vi "02 HEWH Stand Overide.vi"() -> ()   [LabVIEW 2012]
uses:
  EquipReferences.ctl
  HEWH Tank Indicator.ctl
  Intellifaucet/Intellfaucet Mode.ctl
  PowerElements.ctl
  Use Modes.ctl
  <vilib>/Platform/fileVersionInfo.llb/FileVersionInformation.ctl
  GEA2/HEWH_Mode.ctl
  ValveBankPositions.ctl
  ChannelSettings.ctl
  Global HEWH.vi
  <vilib>/Utility/file.llb/Write To Spreadsheet File (string).vi
panel:
  in  "GEA2 Max Retry":i32
  in  "Valve Set D":T1
  in  "Valve Set C":T1
  in  "Valve Set B":T1
  in  "Valve Set A":T1
  out "Source Array":string[](array[string])
  out "Pannel List":string[](array[string])
  in  "GEA2?":bool=TRUE
  out "Data Array":string[][](array[string])
  out "FileVersionInfo Out":T2
  out "Computer Name":string
  out "Label Array":string[](array[string])
  out "Chanel List":string
  in  "Serial Data In":string
  out "RLT":bool
  in  "Out VLV D":enum8{"CLOSE", "OPEN"}(ring)=enum."OPEN"
  in  "Drain VLV D":enum8{"OPEN", "CLOSE"}(ring)=enum."CLOSE"
  in  "In VLV D":enum8{"OPEN", "CLOSE"}(ring)=enum."CLOSE"
  in  "Out VLV C":enum8{"CLOSE", "OPEN"}(ring)=enum."OPEN"
  in  "Drain VLV C":enum8{"OPEN", "CLOSE"}(ring)=enum."CLOSE"
  in  "In VLV C":enum8{"OPEN", "CLOSE"}(ring)=enum."CLOSE"
  in  "Out VLV B":enum8{"CLOSE", "OPEN"}(ring)=enum."OPEN"
  in  "Drain VLV B":enum8{"OPEN", "CLOSE"}(ring)=enum."CLOSE"
  in  "In VLV B":enum8{"OPEN", "CLOSE"}(ring)=enum."CLOSE"
  out "IP Add":string
  out "BUG array":string[](array[string])
  in  "Data File Directory":path=path "c:/data"
  out "Ver.":string="Development"
  in  "COM Port":refnum<visa-resource-name>="COM3"
  in  "DRM Mode Setting":T3=3 items=["CRITICAL", "HIGH", "MEDIUM", "Normal"]
  in  "Equipment":T4={"COM Port"="COM3", "MW100"="MW100", "AG34970"="A-34972A", "Chamber"="WT500"}
  out "MW100":refnum<visa-resource-name>
  out "Local?":bool=TRUE
  in  "Help":bool
  in  "Out VLV":enum8{"CLOSE", "OPEN"}(ring)=enum."OPEN"
  in  "Drain VLV":enum8{"OPEN", "CLOSE"}(ring)=enum."CLOSE"
  in  "In VLV":enum8{"OPEN", "CLOSE"}(ring)=enum."CLOSE"
  out "Error Out":errorcluster
  out "Ready":bool
  in  "Stop Test":bool
  in  "HEWH Power":bool
  in  "Semiphore":T5=refnum
  in  "Safe Mode":bool=TRUE
  in  "Expansion Tank?":bool=TRUE
  in  "IF Stop":bool
  in  "IF Start":bool
  in  "IFaucet Driver":bool
  in  "Percent Flow":dbl(slide)=100.0 scale=0.0..100.0
  in  "Temperature(F)":dbl(slide)=58.0 scale=40.0..120.0
  in  "Mode":T6
  in  "Error In":errorcluster
  out "Update Mode":bool=TRUE
  in  "SetPoint":u8=130
  out "Stop Err":errorcluster
  out "IF Error":errorcluster
  out "kW":dbl
  in  "GEA2 Mode Read":T7=enum."Vacation"
  out "Serial Port Error":errorcluster
  in  "Reset Count":bool
  in  "P-H":bool
  out "Use Agilent?":bool
  out "Gather Data Error":errorcluster
  out "Header?":bool=TRUE
  out "Voltage Reading":dbl=240.0
  in  "Sample Period (S)":dbl=10.0
  out "POWER":T8
  out "Serial Port Available?":bool=TRUE
  in  "Write To File":bool
  out "file path (dialog if empty)":path=path "c:/data/20110112-2122_HEWH-MAN_OV.csv"
  out "WriteDataCount":i32
  out "DATA - Label, Value, Source":string[][](array[string])
  out "Tank Display":T9 {"TC6" format="%.2g"; "TIN" format="%.2g"; "TOUT" format="%.2g"; "Mean" format="%.2f"; "Std Dev" format="%.2f"; "TC5" format="%.2g"; "TC4" format="%.2g"; "TC3" format="%.2g"; "TC2" format="%.2g"; "TC1" format="%.2g"}
  in  "Termperature":dbl=58.0 format="%_6g"
  in  "Read Flow":bool=TRUE
  out "Pulse":i32
  in  "Flow Totalizer Control":bool=TRUE
  out "Dispensed":dbl
  out "ToutMin":dbl
  out "ToutMax":dbl
  in  "Gallon Target":dbl=10.72
  in  "GPM Target":dbl=3.0
  in  "Dispense":bool
  out "LBS":dbl
  in  "Reset Totalizer":bool
  out "Gallons":dbl
  out "Flow Meter":dbl(graph)
  # "HEWH Test Stand Overide"
  # "Intellifaucet Control"
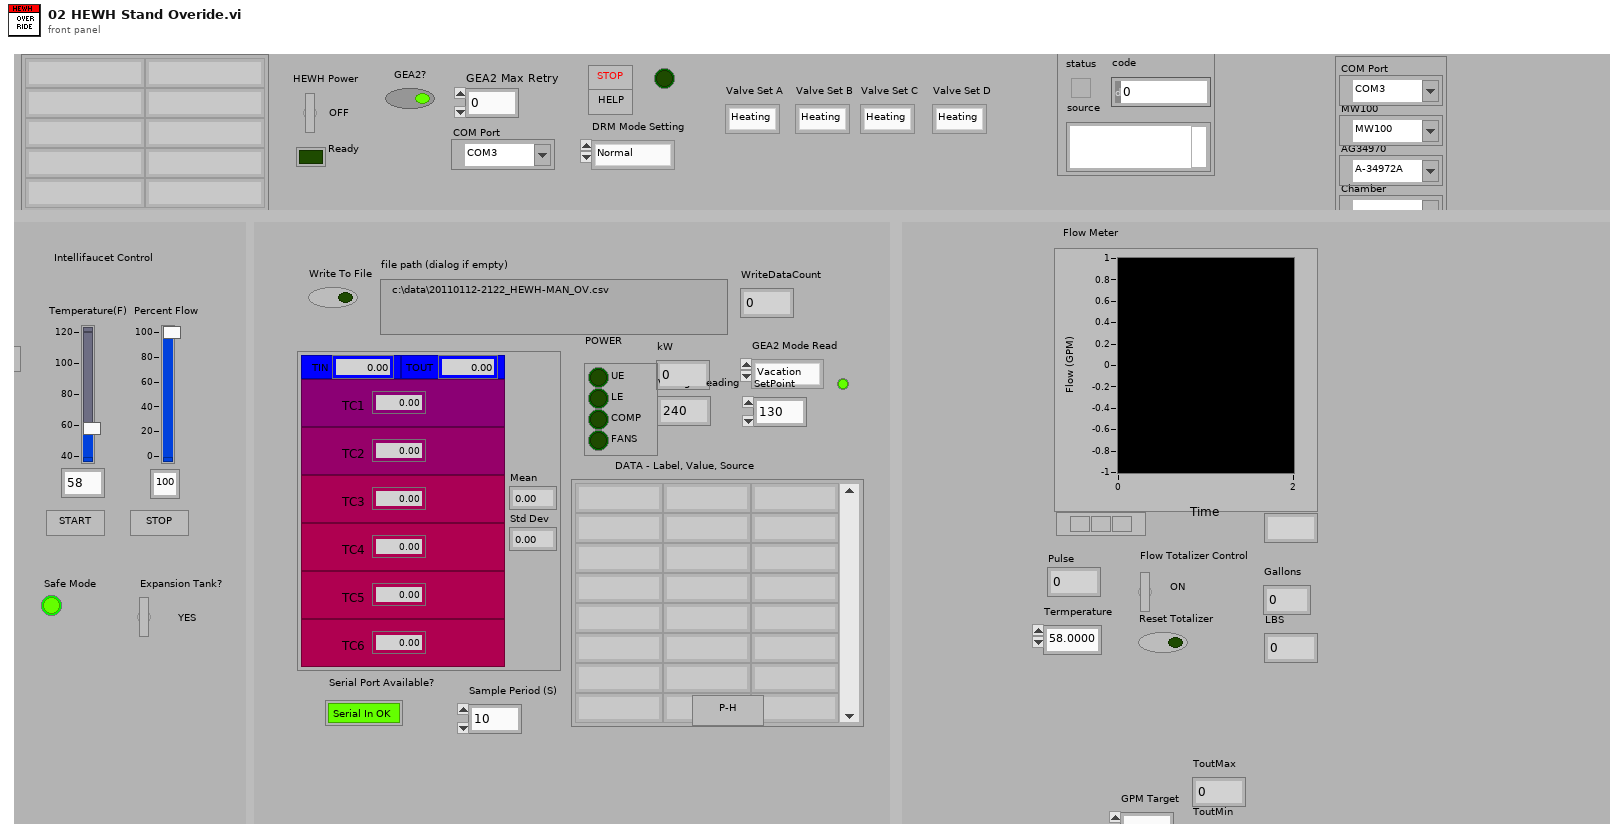
[diagram p1: front panel]
types:
  T1 = typedef "ValveBankPositions.ctl" = enum16{"Heating", "Purge", "Resting", "Draw"}
  T2 = typedef "FileVersionInformation.ctl" = cluster{"FileVersion":string, "ProductName":string, "InternalName":string, "CompanyName":string, "LegalCopyright":string, "FileDescription":string}
  T3 = typedef "Use Modes.ctl" = u16
  T4 = typedef "EquipReferences.ctl" = cluster{"COM Port":refnum<visa-resource-name>, "MW100":refnum<visa-resource-name>, "AG34970":refnum<visa-resource-name>, "Chamber":refnum<visa-resource-name>}
  T5 = typedef "Semaphore RefNum" = refnum<k1>
  T6 = typedef "Intellfaucet Mode.ctl" = enum16{"Adjust Temp", "Adjust Flow", "Start Flow", "Stop Flow"}
  T7 = typedef "HEWH_Mode.ctl" = enum16{"Hybrid", "StdElectric", "eHeat", "HighDemand", "Vacation"}
  T8 = typedef "PowerElements.ctl" = cluster{"UE":bool, "LE":bool, "COMP":bool, "FANS":bool}
  T9 = typedef "HEWH Tank Indicator.ctl" = cluster{"TC1-D":bool, "TC2-D":bool, "TC3-D":bool, "TC4-D":bool, "TC5-D":bool, "RTD_IN":bool, "RTDOUT":bool, "TC1":dbl, "TC2":dbl, "TC3":dbl, "TC4":dbl, "TC5":dbl, "TIN":dbl, "TOUT":dbl, "Std Dev":dbl, "Mean":dbl, "TC6-D":bool, "TC6":dbl}
  T10 = typedef "ChannelSettings.ctl" = u32
  T11 = enum16{"Computation Start", "Computation stop", "Reset Computation", "Clear Computation"}
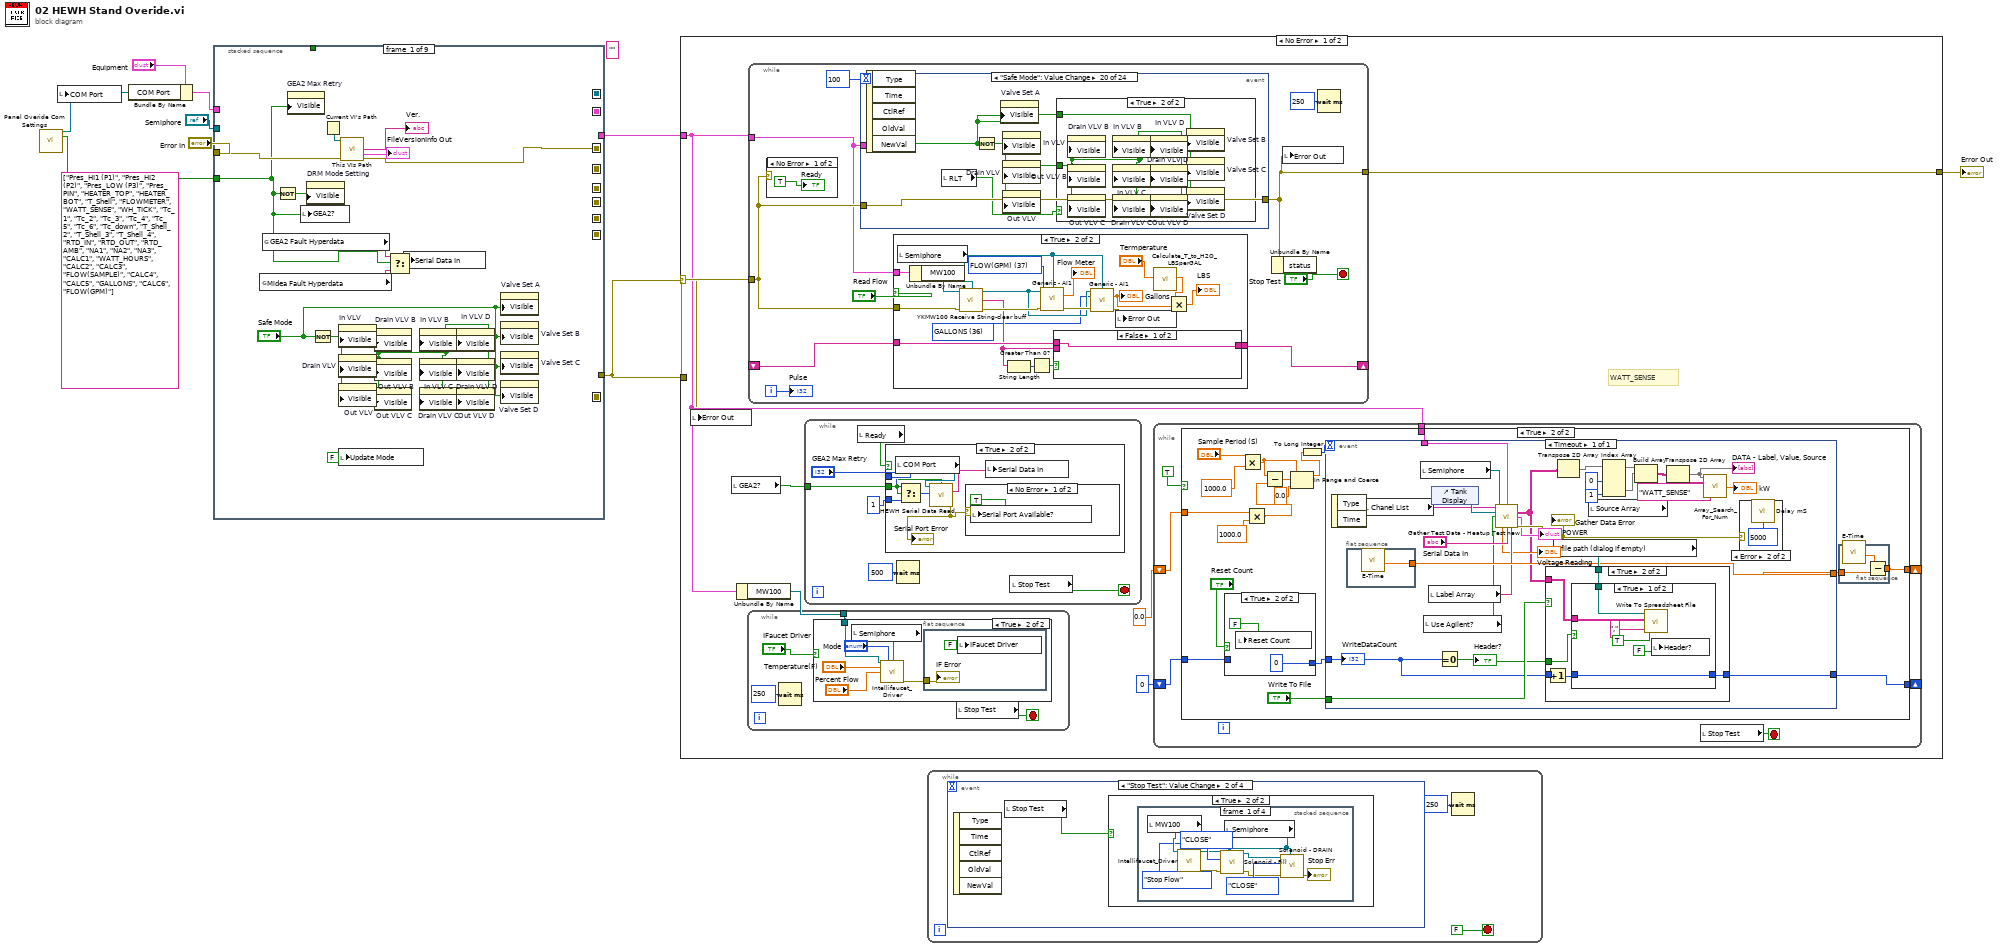
[diagram p0: block diagram]
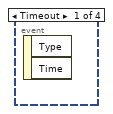
[diagram p2: hidden frame]
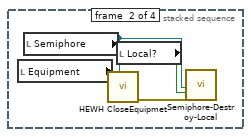
[diagram p4: hidden frame]
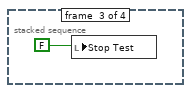
[diagram p5: hidden frame]
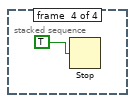
[diagram p6: hidden frame]
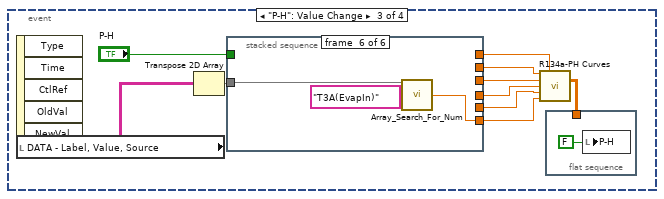
[diagram p7: hidden frame]
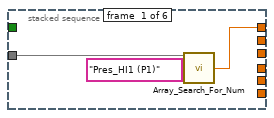
[diagram p8: hidden frame]
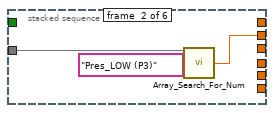
[diagram p9: hidden frame]
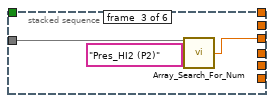
[diagram p10: hidden frame]
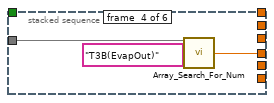
[diagram p11: hidden frame]
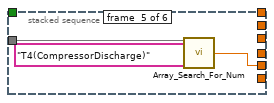
[diagram p12: hidden frame]
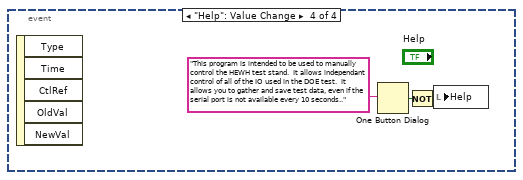
[diagram p13: hidden frame]
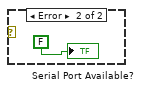
[diagram p15: hidden frame]
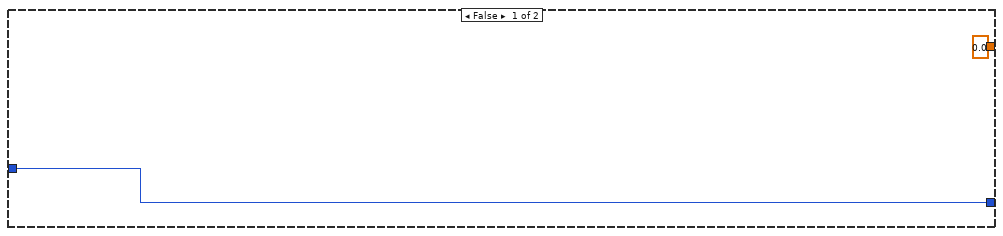
[diagram p17: hidden frame]
diagram:
  (unwired) "" ("Label.Text")
  (unwired) string[] ["Pres_HI1 (P1)", "Pres_HI2 (P2)", "Pres_LOW (P3)", "Pres_PIN", "HEATER_TOP", "HEATER_BOT", "T_Shell", "FLOWMETER", "WATT_SENSE", "WH_TICK", "Tc_1", "Tc_2", "Tc_3", "Tc_4", "Tc_5", "Tc_6", "Tc_down", "T_Shell_2", "T_Shell_3", "T_Shell_4", "RTD_IN", "RTD_OUT", "RTD_AMB", "NA1", "NA2", "NA3", "CALC1", "WATT_HOURS", "CALC2", "CALC3", "FLOW(SAMPLE)", "CALC4", "CALC5", "GALLONS", "CALC6", "FLOW(GPM)"] ("output array")
  n1 = call "Panel Overide Com Settings.vi"() -> ("COM Port Out"=w1:refnum<visa-resource-name>, "GEA2 HyperData Out"=w2:bool)  [unwired: 14 in]
  n2 = local write "COM Port"(w1) -> ()
  n3 = Bundle By Name(cluster="Equipment", "COM Port"=w1) -> (w4:T4)
  n4 = stacked-sequence {
    seq-local: [_ _ w45 _ _ _ _ _ _] -> [_ _ _ w77 _ _ _ _ _]
    seq-local: [_ _ w41 _ _ _ _ _ _] -> [_ _ _ w64 w93 w115 w129 _ _]
    seq-local: [w19 _ _ _ _ _ _ _ _] -> [_ w27 _ _ _ _ _ _ _]
    seq-local: [_ w34 _ _ _ _ _ _ _] -> [_ _ w38 _ _ _ _ _ _]
    seq-local: [_ _ _ w61 _ _ _ _ _] -> [_ _ _ _ w88 _ _ _ _]
    seq-local: [_ _ _ _ w89 _ _ _ _] -> [_ _ _ _ _ w107 _ _ _]
    seq-local: [_ _ _ _ _ w108 _ _ _] -> [_ _ _ _ _ _ w130 _ _]
    seq-local: [_ _ _ _ _ _ w132 _ _] -> [_ _ _ _ _ _ _ w158 _]
    seq-local: [_ _ w37 _ _ _ _ _ _] -> [_ _ _ w60 w87 w106 w128 w157 w175]
    tunnel: "Error In" -> [w20 _ _ _ _ _ _ _ _]
    tunnel: w4 -> [_ _ w46 _ _ _ _ _ _]
    tunnel: [_ _ w37 _ _ _ _ _ _] -> w8
    tunnel: [_ _ _ _ _ _ _ w155 _] -> w7
    tunnel: [_ _ w40 _ _ _ _ _ _] -> _
    tunnel: "Semiphore" -> [_ _ w43 _ _ _ _ _ _]
    tunnel: w2 -> [w10 _ _ _ _ _ _ _ _]
    frame #0 {
      n5 = global read "Global HEWH.vi" "Midea Fault Hyperdata"() -> (w15:string)
      n6 = global read "Global HEWH.vi" "GEA2 Fault Hyperdata"() -> (w16:string)
      n7 = Not(x=w10) -> (.not. x?=w11:bool)
      n8 = property on="GEA2 Max Retry" class="DigNum (strict)"("Visible"=w10) -> ()  [unwired: 2 in, 2 out]
      n9 = local write "GEA2?"(w10) -> ()
      n10 = property on="DRM Mode Setting" class="Ring (strict)"("Visible"=w11) -> ()  [unwired: 2 in, 2 out]
      n11 = Not(x="Safe Mode") -> (.not. x?=w14:bool)
      n12 = Current VI's Path() -> (path=w22:path)
      n13 = local write "Update Mode"(FALSE ("Update Mode")) -> ()
      n14 = property on="In VLV" class="Enum (strict)"("Visible"=w14) -> ()  [unwired: 2 in, 2 out]
      n15 = property on="Drain VLV" class="Enum (strict)"("Visible"=w14) -> ()  [unwired: 2 in, 2 out]
      n16 = property on="Out VLV" class="Enum (strict)"("Visible"=w14) -> ()  [unwired: 2 in, 2 out]
      n17 = call "This VIs Path.vi"("path"=w22, "error in (no error)"=w20) -> ("File Version Info"=→"Ver.":string, "FileVersionInfo Out"=→"FileVersionInfo Out":T2, "error out"=w19:errorcluster)  [unwired: 9 in, 2 out]
      n18 = property on="Drain VLV B" class="Enum (strict)"("Visible"=w14) -> ()  [unwired: 2 in, 2 out]
      n19 = property on="Out VLV B" class="Enum (strict)"("Visible"=w14) -> ()  [unwired: 2 in, 2 out]
      n20 = property on="Out VLV C" class="Enum (strict)"("Visible"=w14) -> ()  [unwired: 2 in, 2 out]
      n21 = Select(t=w16, s=w10, f=w15) -> (s? t:f=w17:string)
      n22 = local write "Serial Data In"(w17) -> ()
      n23 = property on="In VLV B" class="Enum (strict)"("Visible"=w14) -> ()  [unwired: 2 in, 2 out]
      n24 = property on="In VLV C" class="Enum (strict)"("Visible"=w14) -> ()  [unwired: 2 in, 2 out]
      n25 = property on="Drain VLV C" class="Enum (strict)"("Visible"=w14) -> ()  [unwired: 2 in, 2 out]
      n26 = property on="In VLV D" class="Enum (strict)"("Visible"=w14) -> ()  [unwired: 2 in, 2 out]
      n27 = property on="Drain VLV D" class="Enum (strict)"("Visible"=w14) -> ()  [unwired: 2 in, 2 out]
      n28 = property on="Out VLV D" class="Enum (strict)"("Visible"=w14) -> ()  [unwired: 2 in, 2 out]
      n29 = property on="Valve Set A" class="Enum (strict)"("Visible"="Safe Mode") -> ()  [unwired: 2 in, 2 out]
      n30 = property on="Valve Set B" class="Enum (strict)"("Visible"="Safe Mode") -> ()  [unwired: 2 in, 2 out]
      n31 = property on="Valve Set C" class="Enum (strict)"("Visible"="Safe Mode") -> ()  [unwired: 2 in, 2 out]
      n32 = property on="Valve Set D" class="Enum (strict)"("Visible"="Safe Mode") -> ()  [unwired: 2 in, 2 out]
    }
    frame #1 {
      w33 = TRUE ("Reset")
      n33 = local read "FileVersionInfo Out"() -> (w31:T2)
      n34 = call "IP and Computer Name.vi"() -> ("Computer Name"=w32:string)  [unwired: 10 in, 1 out]
      "Computer Name" <- w32
      n35 = Unbundle By Name(w31) -> ("FileVersion"=w30:string)  [unwired: 1 out]
      n36 = call "Data_File_Init.vi"("Data File Directory"="Data File Directory", "Test_Name In:"="MANOV", "Version In:"=w30, "Computer Name In:"=w32, "error in (no error)"=w27, "File Extension:"="csv") -> ("FileName"=→"file path (dialog if empty)":path, "Data Array"=→"Data Array":string[][], "error out"=w28:errorcluster)  [unwired: 7 in]
      n37 = local write "Header?"(w33) -> ()
      n38 = call "E-Time.vi"("error in (no error)"=w28, "Reset"=w33) -> ("error out"=w34:errorcluster)  [unwired: 7 in, 2 out]
    }
    frame #2 {
      w36 = FALSE ("Visible")
      n39 = call "Semiphore-Create-Local.vi"("Semiphore"=w43, "error in (no error)"=w38, "name (unnamed)"="MW100") -> ("semaphore"=w41:T5, "Local?"=w40:bool, "error out"=w44:errorcluster)  [unwired: 14 in]
      "Local?" <- w40
      n40 = local write "Dispense"(w36) -> ()
      n41 = property on="BUG array" class="Arr (strict)"("Visible"=w36) -> ()  [unwired: 2 in, 2 out]
      n42 = local write "P-H"(w36) -> ()
      n43 = local write "Semiphore"(w41) -> ()
      n44 = case shown="True" TRUE {
        tunnel: w44 -> [w48 w56]
        tunnel: [w48 w55] -> w45
        tunnel: w46 -> [w47 w54]
        tunnel: [w47 w49] -> w37
        tunnel: w41 -> [_ w52]
        frame False {
        }
        frame True {
          n45 = call "HEWH InitializeEquipmet.vi"("Semiphore"=w52, "Error In"=w56, "Equipment"=w54) -> ("Error Out"=w55:errorcluster, "LAN IP Address"=→"IP Add":string, "Equipment Out"=w49:T4)  [unwired: 5 in, 1 out]
          n46 = local write "Ready"(FALSE ("Ready")) -> ()
          n47 = Unbundle(w49) -> ("MW100"=→"MW100":refnum<visa-resource-name>)  [unwired: 3 out]
          n48 = local write "Equipment"(w49) -> ()
        }
      }
      n49 = local write "Reset Totalizer"(w36) -> ()
      "Tank Display" <- T9 {"TC1-D"=FALSE, "TC2-D"=FALSE, "TC3-D"=FALSE, "TC4-D"=FALSE, "TC5-D"=FALSE, "RTD_IN"=FALSE, "RTDOUT"=FALSE, "TC1"=0.0, "TC2"=0.0, "TC3"=0.0, "TC4"=0.0, "TC5"=0.0, "TIN"=0.0, "TOUT"=0.0, "Std Dev"=0.0, "Mean"=0.0, "TC6-D"=FALSE, "TC6"=0.0} ("Tank Display")
    }
    frame #3 {
      w65 = FALSE ("Stop Test")
      w69 = T10 30 items=["4-20_OUT", "Pres_HI1", "Pres_HI2", "Pres_LOW", "Pres_PIN", "HEATER_TOP", "HEATER_BOT", "T_Shell", "FLOWMETER", "WATT_SENSE", "WH_TICK", "Tc_1", "Tc_2", "Tc_3", "Tc_4", "Tc_5", "Tc_6", "Tc_down", "T_Shell_2", "T_Shell_3", "T_Shell_4", "RTD_IN", "RTD_OUT", "RTD_AMB", "INTF_TEMPFLO", "INTF_READY", "INTF_START", "INTF_STOP", "DRM_LOW", "DRM_HIGH", "PWR_MAIN", "VLV_DUMP", "VLV_OUT", "VLV_IN", "WATT_HOURS", "FLOW(SAMPLE)", "GALLONS", "FLOW(GPM)"] ("Channel_Enum")
      w70 = T10 33 items=["4-20_OUT", "Pres_HI1", "Pres_HI2", "Pres_LOW", "Pres_PIN", "HEATER_TOP", "HEATER_BOT", "T_Shell", "FLOWMETER", "WATT_SENSE", "WH_TICK", "Tc_1", "Tc_2", "Tc_3", "Tc_4", "Tc_5", "Tc_6", "Tc_down", "T_Shell_2", "T_Shell_3", "T_Shell_4", "RTD_IN", "RTD_OUT", "RTD_AMB", "INTF_TEMPFLO", "INTF_READY", "INTF_START", "INTF_STOP", "DRM_LOW", "DRM_HIGH", "PWR_MAIN", "VLV_DUMP", "VLV_OUT", "VLV_IN", "WATT_HOURS", "FLOW(SAMPLE)", "GALLONS", "FLOW(GPM)"] ("Channel_Enum")
      w71 = T10 32 items=["4-20_OUT", "Pres_HI1", "Pres_HI2", "Pres_LOW", "Pres_PIN", "HEATER_TOP", "HEATER_BOT", "T_Shell", "FLOWMETER", "WATT_SENSE", "WH_TICK", "Tc_1", "Tc_2", "Tc_3", "Tc_4", "Tc_5", "Tc_6", "Tc_down", "T_Shell_2", "T_Shell_3", "T_Shell_4", "RTD_IN", "RTD_OUT", "RTD_AMB", "INTF_TEMPFLO", "INTF_READY", "INTF_START", "INTF_STOP", "DRM_LOW", "DRM_HIGH", "PWR_MAIN", "VLV_DUMP", "VLV_OUT", "VLV_IN", "WATT_HOURS", "FLOW(SAMPLE)", "GALLONS", "FLOW(GPM)"] ("Channel_Enum")
      w73 = T10 31 items=["4-20_OUT", "Pres_HI1", "Pres_HI2", "Pres_LOW", "Pres_PIN", "HEATER_TOP", "HEATER_BOT", "T_Shell", "FLOWMETER", "WATT_SENSE", "WH_TICK", "Tc_1", "Tc_2", "Tc_3", "Tc_4", "Tc_5", "Tc_6", "Tc_down", "T_Shell_2", "T_Shell_3", "T_Shell_4", "RTD_IN", "RTD_OUT", "RTD_AMB", "INTF_TEMPFLO", "INTF_READY", "INTF_START", "INTF_STOP", "DRM_LOW", "DRM_HIGH", "PWR_MAIN", "VLV_DUMP", "VLV_OUT", "VLV_IN", "WATT_HOURS", "FLOW(SAMPLE)", "GALLONS", "FLOW(GPM)"] ("Channel_Enum")
      n50 = local read "Safe Mode"() -> (w58:bool)
      n51 = Unbundle By Name(w60) -> ("MW100"=w72:refnum<visa-resource-name>)
      n52 = local write "IFaucet Driver"(w65) -> ()
      n53 = local write "Stop Test"(w65) -> ()
      n54 = local write "Ready"(w65) -> ()
      n55 = call "YKMW100 VF0 Relay Status.vi"("VISA session"=w72, "Semiphore"=w64, "Channel_Enum"=w69, "error in (no error)"=w77) -> ("Output On"=w62:bool, "DO Card in Slot 5"=w59:bool, "error out"=w76:errorcluster)  [unwired: 8 in, 1 out]
      "RLT" <- w59
      n56 = call "YKMW100 VF0 Relay Status.vi"("VISA session"=w72, "Semiphore"=w64, "Channel_Enum"=w70, "error in (no error)"=w76) -> ("Output On"=w68:bool, "error out"=w75:errorcluster)  [unwired: 8 in, 2 out]
      n57 = call "YKMW100 VF0 Relay Status.vi"("VISA session"=w72, "Semiphore"=w64, "Channel_Enum"=w71, "error in (no error)"=w75) -> ("Output On"=w67:bool, "error out"=w74:errorcluster)  [unwired: 8 in, 2 out]
      n58 = call "YKMW100 VF0 Relay Status.vi"("VISA session"=w72, "Semiphore"=w64, "Channel_Enum"=w73, "error in (no error)"=w74) -> ("Output On"=w66:bool, "error out"=w61:errorcluster)  [unwired: 8 in, 2 out]
      n59 = Not(x=w58) -> (.not. x?=w57:bool)
      n60 = case shown="False" w59 {
        tunnel: w57 -> [w79 _]
        tunnel: w58 -> [w78 _]
        frame True {
          n61 = property on="Drain VLV B" class="Enum (strict)"("Visible"=w79) -> ()  [unwired: 2 in, 2 out]
          n62 = property on="Out VLV B" class="Enum (strict)"("Visible"=w79) -> ()  [unwired: 2 in, 2 out]
          n63 = property on="Out VLV C" class="Enum (strict)"("Visible"=w79) -> ()  [unwired: 2 in, 2 out]
          n64 = property on="In VLV B" class="Enum (strict)"("Visible"=w79) -> ()  [unwired: 2 in, 2 out]
          n65 = property on="In VLV C" class="Enum (strict)"("Visible"=w79) -> ()  [unwired: 2 in, 2 out]
          n66 = property on="Drain VLV C" class="Enum (strict)"("Visible"=w79) -> ()  [unwired: 2 in, 2 out]
          n67 = property on="In VLV D" class="Enum (strict)"("Visible"=w79) -> ()  [unwired: 2 in, 2 out]
          n68 = property on="Drain VLV D" class="Enum (strict)"("Visible"=w79) -> ()  [unwired: 2 in, 2 out]
          n69 = property on="Out VLV D" class="Enum (strict)"("Visible"=w79) -> ()  [unwired: 2 in, 2 out]
          n70 = property on="Valve Set B" class="Enum (strict)"("Visible"=w78) -> ()  [unwired: 2 in, 2 out]
          n71 = property on="Valve Set C" class="Enum (strict)"("Visible"=w78) -> ()  [unwired: 2 in, 2 out]
          n72 = property on="Valve Set D" class="Enum (strict)"("Visible"=w78) -> ()  [unwired: 2 in, 2 out]
        }
        frame False {
          w80 = FALSE ("Visible")
          n73 = property on="Drain VLV B" class="Enum (strict)"("Visible"=w80) -> ()  [unwired: 2 in, 2 out]
          n74 = property on="Out VLV B" class="Enum (strict)"("Visible"=w80) -> ()  [unwired: 2 in, 2 out]
          n75 = property on="Out VLV C" class="Enum (strict)"("Visible"=w80) -> ()  [unwired: 2 in, 2 out]
          n76 = property on="In VLV B" class="Enum (strict)"("Visible"=w80) -> ()  [unwired: 2 in, 2 out]
          n77 = property on="In VLV C" class="Enum (strict)"("Visible"=w80) -> ()  [unwired: 2 in, 2 out]
          n78 = property on="Drain VLV C" class="Enum (strict)"("Visible"=w80) -> ()  [unwired: 2 in, 2 out]
          n79 = property on="In VLV D" class="Enum (strict)"("Visible"=w80) -> ()  [unwired: 2 in, 2 out]
          n80 = property on="Drain VLV D" class="Enum (strict)"("Visible"=w80) -> ()  [unwired: 2 in, 2 out]
          n81 = property on="Out VLV D" class="Enum (strict)"("Visible"=w80) -> ()  [unwired: 2 in, 2 out]
          n82 = property on="Valve Set B" class="Enum (strict)"("Visible"=w80) -> ()  [unwired: 2 in, 2 out]
          n83 = property on="Valve Set C" class="Enum (strict)"("Visible"=w80) -> ()  [unwired: 2 in, 2 out]
          n84 = property on="Valve Set D" class="Enum (strict)"("Visible"=w80) -> ()  [unwired: 2 in, 2 out]
        }
      }
      n85 = Not(x=w62) -> (.not. x?=w63:bool)
      n86 = case shown="False" w68 {
        frame True {
          n87 = local write "In VLV"(enum8{"OPEN", "CLOSE"}."CLOSE" ("INPUT VALVE")) -> ()
        }
        frame False {
          n88 = local write "In VLV"(enum8{"OPEN", "CLOSE"}."OPEN" ("INPUT VALVE")) -> ()
        }
      }
      n89 = case shown="False" w66 {
        frame True {
          n90 = local write "Drain VLV"(enum8{"OPEN", "CLOSE"}."OPEN" ("DRAIN VALVE")) -> ()
        }
        frame False {
          n91 = local write "Drain VLV"(enum8{"OPEN", "CLOSE"}."CLOSE" ("DRAIN VALVE")) -> ()
        }
      }
      n92 = case shown="False" w67 {
        frame True {
          n93 = local write "Out VLV"(enum8{"CLOSE", "OPEN"}."CLOSE" ("VALVE OUT")) -> ()
        }
        frame False {
          n94 = local write "Out VLV"(enum8{"CLOSE", "OPEN"}."OPEN" ("VALVE OUT")) -> ()
        }
      }
      n95 = local write "HEWH Power"(w63) -> ()
      n96 = property on="RLT" class="Bool (strict)"("Val(Sgnl)"=w59) -> ()  [unwired: 2 in, 2 out]
    }
    frame #4 {
      w92 = T10 41 items=["4-20_OUT", "Pres_HI1", "Pres_HI2", "Pres_LOW", "Pres_PIN", "HEATER_TOP", "HEATER_BOT", "T_Shell", "FLOWMETER", "WATT_SENSE", "WH_TICK", "Tc_1", "Tc_2", "Tc_3", "Tc_4", "Tc_5", "Tc_6", "Tc_down", "T_Shell_2", "T_Shell_3", "T_Shell_4", "RTD_IN", "RTD_OUT", "RTD_AMB", "INTF_TEMPFLO", "INTF_READY", "INTF_START", "INTF_STOP", "DRM_LOW", "DRM_HIGH", "PWR_MAIN", "VLV_DUMP", "VLV_OUT", "VLV_IN", "WATT_HOURS", "FLOW(SAMPLE)", "GALLONS", "FLOW(GPM)", "FLOW_CALC_GAIN", "FLOW_CALC_OFFSET", "FLOW_CALC_THRESHOLD", "VLV_DUMP_2", "VLV_OUT_2", "VLV_IN_2", "VLV_DUMP_3", "VLV_OUT_3", "VLV_IN_3", "VLV_DUMP_4", "VLV_OUT_4", "VLV_IN_4"] ("Channel_Enum")
      w91 = T10 42 items=["4-20_OUT", "Pres_HI1", "Pres_HI2", "Pres_LOW", "Pres_PIN", "HEATER_TOP", "HEATER_BOT", "T_Shell", "FLOWMETER", "WATT_SENSE", "WH_TICK", "Tc_1", "Tc_2", "Tc_3", "Tc_4", "Tc_5", "Tc_6", "Tc_down", "T_Shell_2", "T_Shell_3", "T_Shell_4", "RTD_IN", "RTD_OUT", "RTD_AMB", "INTF_TEMPFLO", "INTF_READY", "INTF_START", "INTF_STOP", "DRM_LOW", "DRM_HIGH", "PWR_MAIN", "VLV_DUMP", "VLV_OUT", "VLV_IN", "WATT_HOURS", "FLOW(SAMPLE)", "GALLONS", "FLOW(GPM)", "FLOW_CALC_GAIN", "FLOW_CALC_OFFSET", "FLOW_CALC_THRESHOLD", "VLV_DUMP_2", "VLV_OUT_2", "VLV_IN_2", "VLV_DUMP_3", "VLV_OUT_3", "VLV_IN_3", "VLV_DUMP_4", "VLV_OUT_4", "VLV_IN_4"] ("Channel_Enum")
      w90 = T10 43 items=["4-20_OUT", "Pres_HI1", "Pres_HI2", "Pres_LOW", "Pres_PIN", "HEATER_TOP", "HEATER_BOT", "T_Shell", "FLOWMETER", "WATT_SENSE", "WH_TICK", "Tc_1", "Tc_2", "Tc_3", "Tc_4", "Tc_5", "Tc_6", "Tc_down", "T_Shell_2", "T_Shell_3", "T_Shell_4", "RTD_IN", "RTD_OUT", "RTD_AMB", "INTF_TEMPFLO", "INTF_READY", "INTF_START", "INTF_STOP", "DRM_LOW", "DRM_HIGH", "PWR_MAIN", "VLV_DUMP", "VLV_OUT", "VLV_IN", "WATT_HOURS", "FLOW(SAMPLE)", "GALLONS", "FLOW(GPM)", "FLOW_CALC_GAIN", "FLOW_CALC_OFFSET", "FLOW_CALC_THRESHOLD", "VLV_DUMP_2", "VLV_OUT_2", "VLV_IN_2", "VLV_DUMP_3", "VLV_OUT_3", "VLV_IN_3", "VLV_DUMP_4", "VLV_OUT_4", "VLV_IN_4"] ("Channel_Enum")
      n97 = Unbundle By Name(w87) -> ("MW100"=w97:refnum<visa-resource-name>)
      n98 = call "YKMW100 VF0 Relay Status.vi"("VISA session"=w97, "Semiphore"=w93, "Channel_Enum"=w90, "error in (no error)"=w88) -> ("Output On"=w96:bool, "error out"=w99:errorcluster)  [unwired: 8 in, 2 out]
      n99 = call "YKMW100 VF0 Relay Status.vi"("VISA session"=w97, "Semiphore"=w93, "Channel_Enum"=w91, "error in (no error)"=w99) -> ("Output On"=w95:bool, "error out"=w98:errorcluster)  [unwired: 8 in, 2 out]
      n100 = call "YKMW100 VF0 Relay Status.vi"("VISA session"=w97, "Semiphore"=w93, "Channel_Enum"=w92, "error in (no error)"=w98) -> ("Output On"=w94:bool, "error out"=w89:errorcluster)  [unwired: 8 in, 2 out]
      n101 = case shown="True" w94 {
        frame True {
          n102 = local write "Drain VLV B"(enum8{"OPEN", "CLOSE"}."OPEN" ("DRAIN VALVE")) -> ()
        }
        frame False {
          n103 = local write "Drain VLV B"(enum8{"OPEN", "CLOSE"}."CLOSE" ("DRAIN VALVE")) -> ()
        }
      }
      n104 = case shown="False" w96 {
        frame True {
          n105 = local write "In VLV B"(enum8{"OPEN", "CLOSE"}."CLOSE" ("INPUT VALVE")) -> ()
        }
        frame False {
          n106 = local write "In VLV B"(enum8{"OPEN", "CLOSE"}."OPEN" ("INPUT VALVE")) -> ()
        }
      }
      n107 = case shown="True" w95 {
        frame True {
          n108 = local write "Out VLV B"(enum8{"CLOSE", "OPEN"}."CLOSE" ("VALVE OUT")) -> ()
        }
        frame False {
          n109 = local write "Out VLV B"(enum8{"CLOSE", "OPEN"}."OPEN" ("VALVE OUT")) -> ()
        }
      }
    }
    frame #5 {
      w114 = T10 44 items=["4-20_OUT", "Pres_HI1", "Pres_HI2", "Pres_LOW", "Pres_PIN", "HEATER_TOP", "HEATER_BOT", "T_Shell", "FLOWMETER", "WATT_SENSE", "WH_TICK", "Tc_1", "Tc_2", "Tc_3", "Tc_4", "Tc_5", "Tc_6", "Tc_down", "T_Shell_2", "T_Shell_3", "T_Shell_4", "RTD_IN", "RTD_OUT", "RTD_AMB", "INTF_TEMPFLO", "INTF_READY", "INTF_START", "INTF_STOP", "DRM_LOW", "DRM_HIGH", "PWR_MAIN", "VLV_DUMP", "VLV_OUT", "VLV_IN", "WATT_HOURS", "FLOW(SAMPLE)", "GALLONS", "FLOW(GPM)", "FLOW_CALC_GAIN", "FLOW_CALC_OFFSET", "FLOW_CALC_THRESHOLD", "VLV_DUMP_2", "VLV_OUT_2", "VLV_IN_2", "VLV_DUMP_3", "VLV_OUT_3", "VLV_IN_3", "VLV_DUMP_4", "VLV_OUT_4", "VLV_IN_4"] ("Channel_Enum")
      w113 = T10 45 items=["4-20_OUT", "Pres_HI1", "Pres_HI2", "Pres_LOW", "Pres_PIN", "HEATER_TOP", "HEATER_BOT", "T_Shell", "FLOWMETER", "WATT_SENSE", "WH_TICK", "Tc_1", "Tc_2", "Tc_3", "Tc_4", "Tc_5", "Tc_6", "Tc_down", "T_Shell_2", "T_Shell_3", "T_Shell_4", "RTD_IN", "RTD_OUT", "RTD_AMB", "INTF_TEMPFLO", "INTF_READY", "INTF_START", "INTF_STOP", "DRM_LOW", "DRM_HIGH", "PWR_MAIN", "VLV_DUMP", "VLV_OUT", "VLV_IN", "WATT_HOURS", "FLOW(SAMPLE)", "GALLONS", "FLOW(GPM)", "FLOW_CALC_GAIN", "FLOW_CALC_OFFSET", "FLOW_CALC_THRESHOLD", "VLV_DUMP_2", "VLV_OUT_2", "VLV_IN_2", "VLV_DUMP_3", "VLV_OUT_3", "VLV_IN_3", "VLV_DUMP_4", "VLV_OUT_4", "VLV_IN_4"] ("Channel_Enum")
      w112 = T10 46 items=["4-20_OUT", "Pres_HI1", "Pres_HI2", "Pres_LOW", "Pres_PIN", "HEATER_TOP", "HEATER_BOT", "T_Shell", "FLOWMETER", "WATT_SENSE", "WH_TICK", "Tc_1", "Tc_2", "Tc_3", "Tc_4", "Tc_5", "Tc_6", "Tc_down", "T_Shell_2", "T_Shell_3", "T_Shell_4", "RTD_IN", "RTD_OUT", "RTD_AMB", "INTF_TEMPFLO", "INTF_READY", "INTF_START", "INTF_STOP", "DRM_LOW", "DRM_HIGH", "PWR_MAIN", "VLV_DUMP", "VLV_OUT", "VLV_IN", "WATT_HOURS", "FLOW(SAMPLE)", "GALLONS", "FLOW(GPM)", "FLOW_CALC_GAIN", "FLOW_CALC_OFFSET", "FLOW_CALC_THRESHOLD", "VLV_DUMP_2", "VLV_OUT_2", "VLV_IN_2", "VLV_DUMP_3", "VLV_OUT_3", "VLV_IN_3", "VLV_DUMP_4", "VLV_OUT_4", "VLV_IN_4"] ("Channel_Enum")
      n110 = Unbundle By Name(w106) -> ("MW100"=w119:refnum<visa-resource-name>)
      n111 = call "YKMW100 VF0 Relay Status.vi"("VISA session"=w119, "Semiphore"=w115, "Channel_Enum"=w112, "error in (no error)"=w107) -> ("Output On"=w118:bool, "error out"=w121:errorcluster)  [unwired: 8 in, 2 out]
      n112 = call "YKMW100 VF0 Relay Status.vi"("VISA session"=w119, "Semiphore"=w115, "Channel_Enum"=w113, "error in (no error)"=w121) -> ("Output On"=w117:bool, "error out"=w120:errorcluster)  [unwired: 8 in, 2 out]
      n113 = call "YKMW100 VF0 Relay Status.vi"("VISA session"=w119, "Semiphore"=w115, "Channel_Enum"=w114, "error in (no error)"=w120) -> ("Output On"=w116:bool, "error out"=w108:errorcluster)  [unwired: 8 in, 2 out]
      n114 = case shown="True" w118 {
        tunnel: [enum8{"OPEN", "CLOSE"}."CLOSE" ("INPUT VALVE") enum8{"OPEN", "CLOSE"}."OPEN" ("INPUT VALVE")] -> w111
        frame True {
        }
        frame False {
        }
      }
      n115 = case shown="True" w116 {
        tunnel: [enum8{"OPEN", "CLOSE"}."OPEN" ("DRAIN VALVE") enum8{"OPEN", "CLOSE"}."CLOSE" ("DRAIN VALVE")] -> w109
        frame True {
        }
        frame False {
        }
      }
      n116 = case shown="True" w117 {
        tunnel: [enum8{"CLOSE", "OPEN"}."CLOSE" ("VALVE OUT") enum8{"CLOSE", "OPEN"}."OPEN" ("VALVE OUT")] -> w110
        frame True {
        }
        frame False {
        }
      }
      n117 = local write "In VLV C"(w111) -> ()
      n118 = local write "Drain VLV C"(w109) -> ()
      n119 = local write "Out VLV C"(w110) -> ()
    }
    frame #6 {
      w143 = T10 47 items=["4-20_OUT", "Pres_HI1", "Pres_HI2", "Pres_LOW", "Pres_PIN", "HEATER_TOP", "HEATER_BOT", "T_Shell", "FLOWMETER", "WATT_SENSE", "WH_TICK", "Tc_1", "Tc_2", "Tc_3", "Tc_4", "Tc_5", "Tc_6", "Tc_down", "T_Shell_2", "T_Shell_3", "T_Shell_4", "RTD_IN", "RTD_OUT", "RTD_AMB", "INTF_TEMPFLO", "INTF_READY", "INTF_START", "INTF_STOP", "DRM_LOW", "DRM_HIGH", "PWR_MAIN", "VLV_DUMP", "VLV_OUT", "VLV_IN", "WATT_HOURS", "FLOW(SAMPLE)", "GALLONS", "FLOW(GPM)", "FLOW_CALC_GAIN", "FLOW_CALC_OFFSET", "FLOW_CALC_THRESHOLD", "VLV_DUMP_2", "VLV_OUT_2", "VLV_IN_2", "VLV_DUMP_3", "VLV_OUT_3", "VLV_IN_3", "VLV_DUMP_4", "VLV_OUT_4", "VLV_IN_4"] ("Channel_Enum")
      w142 = T10 48 items=["4-20_OUT", "Pres_HI1", "Pres_HI2", "Pres_LOW", "Pres_PIN", "HEATER_TOP", "HEATER_BOT", "T_Shell", "FLOWMETER", "WATT_SENSE", "WH_TICK", "Tc_1", "Tc_2", "Tc_3", "Tc_4", "Tc_5", "Tc_6", "Tc_down", "T_Shell_2", "T_Shell_3", "T_Shell_4", "RTD_IN", "RTD_OUT", "RTD_AMB", "INTF_TEMPFLO", "INTF_READY", "INTF_START", "INTF_STOP", "DRM_LOW", "DRM_HIGH", "PWR_MAIN", "VLV_DUMP", "VLV_OUT", "VLV_IN", "WATT_HOURS", "FLOW(SAMPLE)", "GALLONS", "FLOW(GPM)", "FLOW_CALC_GAIN", "FLOW_CALC_OFFSET", "FLOW_CALC_THRESHOLD", "VLV_DUMP_2", "VLV_OUT_2", "VLV_IN_2", "VLV_DUMP_3", "VLV_OUT_3", "VLV_IN_3", "VLV_DUMP_4", "VLV_OUT_4", "VLV_IN_4"] ("Channel_Enum")
      w141 = T10 49 items=["4-20_OUT", "Pres_HI1", "Pres_HI2", "Pres_LOW", "Pres_PIN", "HEATER_TOP", "HEATER_BOT", "T_Shell", "FLOWMETER", "WATT_SENSE", "WH_TICK", "Tc_1", "Tc_2", "Tc_3", "Tc_4", "Tc_5", "Tc_6", "Tc_down", "T_Shell_2", "T_Shell_3", "T_Shell_4", "RTD_IN", "RTD_OUT", "RTD_AMB", "INTF_TEMPFLO", "INTF_READY", "INTF_START", "INTF_STOP", "DRM_LOW", "DRM_HIGH", "PWR_MAIN", "VLV_DUMP", "VLV_OUT", "VLV_IN", "WATT_HOURS", "FLOW(SAMPLE)", "GALLONS", "FLOW(GPM)", "FLOW_CALC_GAIN", "FLOW_CALC_OFFSET", "FLOW_CALC_THRESHOLD", "VLV_DUMP_2", "VLV_OUT_2", "VLV_IN_2", "VLV_DUMP_3", "VLV_OUT_3", "VLV_IN_3", "VLV_DUMP_4", "VLV_OUT_4", "VLV_IN_4"] ("Channel_Enum")
      n120 = Unbundle By Name(w128) -> ("MW100"=w131:refnum<visa-resource-name>)
      n121 = call "YKMW100 VF0 Relay Status.vi"("VISA session"=w131, "Semiphore"=w129, "Channel_Enum"=w141, "error in (no error)"=w130) -> ("Output On"=w146:bool, "error out"=w148:errorcluster)  [unwired: 8 in, 2 out]
      n122 = call "YKMW100 VF0 Relay Status.vi"("VISA session"=w131, "Semiphore"=w129, "Channel_Enum"=w142, "error in (no error)"=w148) -> ("Output On"=w145:bool, "error out"=w147:errorcluster)  [unwired: 8 in, 2 out]
      n123 = call "YKMW100 VF0 Relay Status.vi"("VISA session"=w131, "Semiphore"=w129, "Channel_Enum"=w143, "error in (no error)"=w147) -> ("Output On"=w144:bool, "error out"=w137:errorcluster)  [unwired: 8 in, 2 out]
      n124 = case shown="True" w146 {
        tunnel: [enum8{"OPEN", "CLOSE"}."CLOSE" ("INPUT VALVE") enum8{"OPEN", "CLOSE"}."OPEN" ("INPUT VALVE")] -> w140
        frame True {
        }
        frame False {
        }
      }
      n125 = case shown="True" w144 {
        tunnel: [enum8{"OPEN", "CLOSE"}."OPEN" ("DRAIN VALVE") enum8{"OPEN", "CLOSE"}."CLOSE" ("DRAIN VALVE")] -> w138
        frame True {
        }
        frame False {
        }
      }
      n126 = case shown="True" w145 {
        tunnel: [enum8{"CLOSE", "OPEN"}."CLOSE" ("VALVE OUT") enum8{"CLOSE", "OPEN"}."OPEN" ("VALVE OUT")] -> w139
        frame True {
        }
        frame False {
        }
      }
      n127 = call "YKMW100 Read Com Register.vi"("VISA session"=w131, "Com Channel (C001)"="C001", "error in (no error)"=w137) -> ("Buffer Value"=w136:string, "error out"=w132:errorcluster)  [unwired: 10 in, 1 out]
      n128 = Equal?(x=w136, y="1" ("Buffer Value")) -> (x = y?=w133:bool)
      n129 = local write "Flow Totalizer Control"(w133) -> ()
      n130 = local write "In VLV D"(w140) -> ()
      n131 = local write "Drain VLV D"(w138) -> ()
      n132 = local write "Out VLV D"(w139) -> ()
    }
    frame #7 {
      w159 = 30.0 ("Percent Flow")
      w160 = 58.0 ("Temperature(F)")
      n133 = local write "Temperature(F)"(w160) -> ()
      n134 = local write "Percent Flow"(w159) -> ()
      n135 = property on="Percent Flow" class="Slide (strict)"("Val(Sgnl)"=w159) -> ()  [unwired: 2 in, 2 out]
      n136 = property on="Temperature(F)" class="Slide (strict)"("Val(Sgnl)"=w160) -> ()  [unwired: 2 in, 2 out]
      n137 = Unbundle By Name(w157) -> ("AG34970"=w156:refnum<visa-resource-name>)
      n138 = case shown="No Error" w158 {
        selector: w158 -> [w168 w170]
        tunnel: [w167 w170] -> w155
        tunnel: w156 -> [w166 _]
        frame No Error {
          n139 = call "HEWH Channel Test Labels.vi"() -> ("Chanel List"=w164:string, "Label List"=→"Label Array":string[], "Pannel List"=→"Pannel List":string[])  [unwired: 13 in]
          "Chanel List" <- w164
          n140 = String Length(string=w164) -> (length=w163:i32)
          n141 = call "Agilent Scan EZ Temperature.vi"("VISA Resource Name"=w166, "Control"=enum16{"Initialize", "Read", "Experiment"}."Initialize", "Channel Input"=w164, "error in (no error)"=w168) -> ("error out"=w167:errorcluster)  [unwired: 8 in, 3 out]
          n142 = Greater Than 0?(x=w163) -> (x > 0?=→"Use Agilent?":bool)
        }
        frame Error {
        }
      }
      n143 = local write "Error Out"(w155) -> ()
    }
    frame #8 {
      n144 = Unbundle By Name(w175) -> ("COM Port"=w176:refnum<visa-resource-name>)
      n145 = local read "GEA2?"() -> (w171:bool)
      n146 = case shown="True" w171 {
        selector: w171 -> [w182 _]
        tunnel: [HEWH_Mode."Vacation" ("Mode Read") w188] -> w178
        tunnel: [FALSE ("ACK") w187] -> w177
        tunnel: w176 -> [_ w186]
        tunnel: [u8 0 ("Current SetPoint") w185] -> w172
        frame False {
          n147 = property on="GEA2 Mode Read" class="Enum (strict)"("Visible"=w182) -> ()  [unwired: 2 in, 2 out]
        }
        frame True {
          n148 = while {
            tunnel: [w198] -> w188
            tunnel: [w189] -> w187
            tunnel: w186 -> [w197]
            tunnel: [w190] -> w185
            i -> [w195]
            stop <- w196 continue-if-true
            n149 = call "GEA2_RQST_STATUS_QUERY.vi"("ComPort"=w197) -> ("Mode"=w198:T7, "Current SetPoint"=w190:u8, "CRC Match"=w189:bool, "Error Out"=w192:errorcluster)  [unwired: 9 in, 2 out]
            n150 = Unbundle By Name(w192) -> ("status"=w191:bool)
            n151 = Less Or Equal?(x=w195, y=5) -> (x <= y?=w193:bool)
            n152 = And(x=w191, y=w193) -> (x .and. y?=w196:bool)
          }
        }
      }
      n153 = property on="Update Mode" class="Bool (strict)"("Visible"=w171) -> ()  [unwired: 2 in, 2 out]
      n154 = property on="GEA2 Mode Read" class="Enum (strict)"("Visible"=w171) -> ()  [unwired: 2 in, 2 out]
      n155 = property on="SetPoint" class="DigNum (strict)"("Visible"=w171) -> ()  [unwired: 2 in, 2 out]
      n156 = local read "Pannel List"() -> (w180:string[])
      n157 = call "HEWH Source String Array.vi"("GEA2 HyperData"=w171, "Pannel List"=w180) -> ("Source Array"=w179:string[])  [unwired: 13 in]
      n158 = local write "Source Array"(w179) -> ()
      n159 = case shown="False" w177 {
        tunnel: w178 -> [_ w202]
        tunnel: [HEWH_Mode."Vacation" ("Mode Read") w202] -> w174
        tunnel: [u8 0 ("Current SetPoint") w201] -> w173
        tunnel: w172 -> [_ w201]
        frame False {
        }
        frame True {
        }
      }
      n160 = local write "SetPoint"(w173) -> ()
      n161 = local write "GEA2 Mode Read"(w174) -> ()
    }
  }
  n162 = case shown="No Error" w7 {
    selector: w7 -> [w206 _]
    tunnel: [w210 w522] -> w3
    tunnel: w7 -> [w209 w522]
    tunnel: w8 -> [w208 _]
    frame No Error {
      # "WATT_SENSE"
      n163 = local write "Error Out"(w206) -> ()
      n164 = local read "GEA2?"() -> (w203:bool)
      n165 = Unbundle By Name(w208) -> ("MW100"=w207:refnum<visa-resource-name>)
      n166 = while {
        tunnel: w207 -> [w227]
        stop <- w228 stop-if-true
        n167 = Wait (ms)(milliseconds to wait=u32 250) -> ()  [unwired: 1 out]
        n168 = case shown="True" "IFaucet Driver" {
          tunnel: w227 -> [_ w231]
          frame False {
          }
          frame True {
            n169 = local read "Semiphore"() -> (w235:T5)
            n170 = call "Intellifaucet_Driver.vi"("VISA session"=w231, "Mode"="Mode", "Semiphore"=w235, "Temperature(F)"="Temperature(F)", "Percent Flow"="Percent Flow") -> ("Error Out"=w230:errorcluster)  [unwired: 9 in, 1 out]
            n171 = flat-sequence {
              tunnel: w230 -> [w236]
              frame #0 {
                n172 = local write "IFaucet Driver"(FALSE ("IFaucet Driver")) -> ()
                "IF Error" <- w236
              }
            }
          }
        }
        n173 = local read "Stop Test"() -> (w228:bool)
      }
      n174 = while {
        tunnel: w209 -> [w324]
        tunnel: [w322] -> w210
        shift-right: [w326] -> _
        shift-left: _ -> [w325]
        tunnel: w208 -> [w323]
        i -> [w327]
        stop <- "Stop Test" stop-if-true
        n175 = case shown="No Error" w324 {
          frame No Error {
            "Ready" <- TRUE
          }
          frame Error {
          }
        }
        n176 = event shown="[19] \"Safe Mode\": Value Change" {
          selector: _ -> [_ _ _ _ _ _ _ _ _ _ _ _ _ _ _ _ _ _ _ _ _ _ _ _]
          dyn-events: _ -> [_ _ _ _ _ _ _ _ _ _ _ _ _ _ _ _ _ _ _ _ _ _ _ _]
          timeout: 100 -> [_ _ _ _ _ _ _ _ _ _ _ _ _ _ _ _ _ _ _ _ _ _ _ _]
          tunnel: w324 -> [w357 w363 w367 _ _ _ _ w401 w419 _ w427 w431 w438 w446 _ w454 w463 w468 w475 w482 w491 _ _ _]
          tunnel: [w357 w359 w368 w372 w379 w386 w393 w400 w411 _ w426 w430 w437 w447 _ w453 w462 w467 w474 w482 w490 w498 w509 w517] -> w322
          tunnel: w323 -> [_ w362 w371 w374 w381 w388 w395 w402 w418 _ w429 w435 w441 w448 w449 w452 w459 w471 w478 _ w492 w501 w512 w520]
          event Timeout {
            n177 = event-data() -> ()  [unwired: 1 in, 2 out]
          }
          event "HEWH Power": Value Change {
            w361 = T10 30 items=["4-20_OUT", "Pres_HI1", "Pres_HI2", "Pres_LOW", "Pres_PIN", "HEATER_TOP", "HEATER_BOT", "T_Shell", "FLOWMETER", "WATT_SENSE", "WH_TICK", "Tc_1", "Tc_2", "Tc_3", "Tc_4", "Tc_5", "Tc_6", "Tc_down", "T_Shell_2", "T_Shell_3", "T_Shell_4", "RTD_IN", "RTD_OUT", "RTD_AMB", "INTF_TEMPFLO", "INTF_READY", "INTF_START", "INTF_STOP", "DRM_LOW", "DRM_HIGH", "PWR_MAIN", "VLV_DUMP", "VLV_OUT", "VLV_IN", "WATT_HOURS", "FLOW(SAMPLE)", "GALLONS", "FLOW(GPM)"] ("Channel_Enum")
            n178 = event-data() -> ()  [unwired: 1 in, 5 out]
            n179 = local read "Semiphore"() -> (w360:T5)
            n180 = Unbundle By Name(w362) -> ("MW100"=w364:refnum<visa-resource-name>)
            n181 = Boolean To (0,1)(Boolean="HEWH Power") -> (0, 1=w365:i16)
            n182 = call "Generic - DO1.vi"("VISA session"=w364, "Semiphore"=w360, "Channel_Enum"=w361, "Relay Status (0:CLOSED)"=w365, "Error In"=w363) -> ("error out"=w359:errorcluster)  [unwired: 9 in, 1 out]
          }
          event "Out VLV": Value Change {
            n183 = event-data() -> ()  [unwired: 1 in, 5 out]
            n184 = Unbundle By Name(w371) -> ("MW100"=w370:refnum<visa-resource-name>)
            n185 = local read "Semiphore"() -> (w369:T5)
            n186 = call "Solenoid - Output_Set COM1 Val.vi"("Semiphore"=w369, "Error In"=w367, "OPEN CLOSE"="Out VLV", "VISA session"=w370) -> ("Error Out"=w368:errorcluster)  [unwired: 6 in, 1 out]
          }
          event Value Change {
            w376 = u16 0 items=["A", "B", "C", "D"] ("Valve Bank")
            n187 = event-data() -> ()  [unwired: 1 in, 5 out]
            n188 = Unbundle By Name(w374) -> ("MW100"=w373:refnum<visa-resource-name>)
            n189 = local read "Semiphore"() -> (w377:T5)
            n190 = call "HEWH Set Valves.vi"("VISA session"=w373, "Valve Bank"=w376, "Semiphore"=w377, "Expansion Tank?"="Expansion Tank?", "Valve Bank Setting"="Valve Set A") -> ("Error Out"=w372:errorcluster)  [unwired: 9 in, 1 out]
          }
          event Value Change {
            w383 = u16 1 items=["A", "B", "C", "D"] ("Valve Bank")
            n191 = event-data() -> ()  [unwired: 1 in, 5 out]
            n192 = Unbundle By Name(w381) -> ("MW100"=w380:refnum<visa-resource-name>)
            n193 = local read "Expansion Tank?"() -> (w382:bool)
            n194 = local read "Semiphore"() -> (w384:T5)
            n195 = call "HEWH Set Valves.vi"("VISA session"=w380, "Valve Bank"=w383, "Semiphore"=w384, "Expansion Tank?"=w382, "Valve Bank Setting"="Valve Set B") -> ("Error Out"=w379:errorcluster)  [unwired: 9 in, 1 out]
          }
          event Value Change {
            w390 = u16 2 items=["A", "B", "C", "D"] ("Valve Bank")
            n196 = event-data() -> ()  [unwired: 1 in, 5 out]
            n197 = Unbundle By Name(w388) -> ("MW100"=w387:refnum<visa-resource-name>)
            n198 = local read "Expansion Tank?"() -> (w389:bool)
            n199 = local read "Semiphore"() -> (w391:T5)
            n200 = call "HEWH Set Valves.vi"("VISA session"=w387, "Valve Bank"=w390, "Semiphore"=w391, "Expansion Tank?"=w389, "Valve Bank Setting"="Valve Set C") -> ("Error Out"=w386:errorcluster)  [unwired: 9 in, 1 out]
          }
          event Value Change {
            w397 = u16 3 items=["A", "B", "C", "D"] ("Valve Bank")
            n201 = event-data() -> ()  [unwired: 1 in, 5 out]
            n202 = Unbundle By Name(w395) -> ("MW100"=w394:refnum<visa-resource-name>)
            n203 = local read "Expansion Tank?"() -> (w396:bool)
            n204 = local read "Semiphore"() -> (w398:T5)
            n205 = call "HEWH Set Valves.vi"("VISA session"=w394, "Valve Bank"=w397, "Semiphore"=w398, "Expansion Tank?"=w396, "Valve Bank Setting"="Valve Set D") -> ("Error Out"=w393:errorcluster)  [unwired: 9 in, 1 out]
          }
          event "Reset Totalizer": Value Change {
            n206 = event-data() -> ()  [unwired: 1 in, 5 out]
            n207 = stacked-sequence {
              tunnel: w402 -> [_ w409]
              tunnel: w401 -> [_ w406]
              tunnel: [_ w404] -> w400
              frame #0 {
                n208 = local write "Reset Totalizer"(FALSE ("Reset Computations")) -> ()
              }
              frame #1 {
                n209 = Unbundle By Name(w409) -> ("MW100"=w408:refnum<visa-resource-name>)
                n210 = local read "Semiphore"() -> (w407:T5)
                n211 = call "YKMW100 Computation Control.vi"("VISA session"=w408, "Semiphore"=w407, "Mode"=T11."Reset Computation", "error in (no error)"=w406) -> ("error out"=w404:errorcluster)  [unwired: 10 in, 1 out]
              }
            }
          }
          event "Dispense": Value Change {
            n212 = event-data() -> ()  [unwired: 1 in, 5 out]
            n213 = control-ref of="Flow Meter"() -> (w410:refnum<vi>)
            n214 = local read "Semiphore"() -> (w417:T5)
            n215 = call "Dispense X Gallon at Y Flowrate.vi"("Gallon Target"="Gallon Target", "Equipment"=w418, "Semiphore"=w417, "GPM Target"="GPM Target", "Error In"=w419, "Ctl Refnum"=w410) -> ("M*(Gallons)"=→"Dispensed":dbl, "ToutMax"=→"ToutMax":dbl, "ToutMin"=→"ToutMin":dbl, "Error Out"=w411:errorcluster)  [unwired: 4 in, 2 out]
            n216 = flat-sequence {
              tunnel: w411 -> [_]
              frame #0 {
                n217 = local write "Dispense"(FALSE ("IF Start")) -> ()
              }
            }
          }
          event "GEA2?": Value Change {
            n218 = event-data() -> ()  [unwired: 1 in, 5 out]
            n219 = local read "Pannel List"() -> (w422:string[])
            n220 = call "HEWH Source String Array.vi"("GEA2 HyperData"="GEA2?", "Pannel List"=w422) -> ("Source Array"=→"Source Array":string[])  [unwired: 13 in]
          }
          event "In VLV": Value Change {
            n221 = event-data() -> ()  [unwired: 1 in, 5 out]
            n222 = Unbundle By Name(w429) -> ("MW100"=w424:refnum<visa-resource-name>)
            n223 = local read "Semiphore"() -> (w425:T5)
            n224 = call "Solenoid - Fill.vi"("Semiphore"=w425, "Error In"=w427, "VALVE OPEN CLOSE"="In VLV", "VISA session"=w424) -> ("Error Out"=w426:errorcluster)  [unwired: 6 in, 1 out]
          }
          event "Drain VLV": Value Change {
            n225 = event-data() -> ()  [unwired: 1 in, 5 out]
            n226 = Unbundle By Name(w435) -> ("MW100"=w433:refnum<visa-resource-name>)
            n227 = local read "Semiphore"() -> (w434:T5)
            n228 = call "Solenoid - DRAIN.vi"("Semiphore"=w434, "Error In"=w431, "VALVE OPEN CLOSE"="Drain VLV", "VISA session"=w433) -> ("Error Out"=w430:errorcluster)  [unwired: 6 in, 1 out]
          }
          event "IF Start": Value Change {
            n229 = event-data() -> ()  [unwired: 1 in, 5 out]
            n230 = Unbundle By Name(w441) -> ("MW100"=w439:refnum<visa-resource-name>)
            n231 = local read "Semiphore"() -> (w440:T5)
            n232 = call "Intellifaucet_Driver.vi"("VISA session"=w439, "Mode"=Intellfaucet_Mode."Start Flow", "Semiphore"=w440, "Error In"=w438) -> ("Error Out"=w437:errorcluster)  [unwired: 10 in, 1 out]
            n233 = flat-sequence {
              tunnel: w437 -> [_]
              frame #0 {
                n234 = local write "IF Start"(FALSE ("IF Start")) -> ()
              }
            }
          }
          event "Flow Totalizer Control": Value Change {
            n235 = event-data() -> ()  [unwired: 1 in, 5 out]
            n236 = Unbundle By Name(w448) -> ("MW100"=w444:refnum<visa-resource-name>)
            n237 = local read "Semiphore"() -> (w443:T5)
            n238 = call "HEWH Totalize Flow Control.vi"("VISA session"=w444, "Semiphore"=w443, "Totalize Flow"="Flow Totalizer Control", "error in (no error)"=w446) -> ("error out"=w447:errorcluster)  [unwired: 10 in, 1 out]
          }
          event "COM Port": Value Change {
            n239 = event-data() -> ("NewVal"=w450:refnum<visa-resource-name>)  [unwired: 1 in, 4 out]
            n240 = Bundle By Name(cluster=w449, "COM Port"=w450) -> ()  [unwired: 1 out]
          }
          event "Temperature(F)": Value Change {
            n241 = event-data() -> ("NewVal"=w456:dbl)  [unwired: 1 in, 4 out]
            n242 = Unbundle By Name(w452) -> ("MW100"=w451:refnum<visa-resource-name>)
            n243 = local read "Semiphore"() -> (w457:T5)
            n244 = call "Intellifaucet_Driver.vi"("VISA session"=w451, "Mode"=Intellfaucet_Mode."Adjust Temp", "Semiphore"=w457, "Temperature(F)"=w456, "Error In"=w454) -> ("Error Out"=w453:errorcluster)  [unwired: 9 in, 1 out]
          }
          event "Percent Flow": Value Change {
            n245 = event-data() -> ("NewVal"=w461:dbl)  [unwired: 1 in, 4 out]
            n246 = Unbundle By Name(w459) -> ("MW100"=w458:refnum<visa-resource-name>)
            n247 = local read "Semiphore"() -> (w465:T5)
            n248 = call "Intellifaucet_Driver.vi"("VISA session"=w458, "Mode"=Intellfaucet_Mode."Adjust Flow", "Semiphore"=w465, "Percent Flow"=w461, "Error In"=w463) -> ("Error Out"=w462:errorcluster)  [unwired: 9 in, 1 out]
            n249 = Wait (ms)(milliseconds to wait=u32 1000) -> ()  [unwired: 1 out]
          }
          event "IF Stop": Value Change {
            n250 = event-data() -> ()  [unwired: 1 in, 5 out]
            n251 = Unbundle By Name(w471) -> ("MW100"=w469:refnum<visa-resource-name>)
            n252 = local read "Semiphore"() -> (w470:T5)
            n253 = call "Intellifaucet_Driver.vi"("VISA session"=w469, "Mode"=Intellfaucet_Mode."Stop Flow", "Semiphore"=w470, "Error In"=w468) -> ("Error Out"=w467:errorcluster)  [unwired: 10 in, 1 out]
            n254 = flat-sequence {
              tunnel: w467 -> [_]
              frame #0 {
                n255 = local write "IF Stop"(FALSE ("IF Start")) -> ()
              }
            }
          }
          event Value Change {
            n256 = event-data() -> ()  [unwired: 1 in, 5 out]
            n257 = Unbundle By Name(w478) -> ("MW100"=w476:refnum<visa-resource-name>)
            n258 = local read "Semiphore"() -> (w477:T5)
            n259 = call "HEWH Set DRM Mode.vi"("MW100"=w476, "Semiphore"=w477, "Mode"="DRM Mode Setting", "error in (no error)"=w475) -> ("error out"=w474:errorcluster)  [unwired: 11 in]
          }
          event "Safe Mode": Value Change {
            n260 = event-data() -> ("NewVal"=w480:bool)  [unwired: 1 in, 4 out]
            n261 = local read "RLT"() -> (w479:bool)
            n262 = Not(x=w480) -> (.not. x?=w481:bool)
            n263 = property on="Valve Set A" class="Enum (strict)"("Visible"=w480) -> ()  [unwired: 2 in, 2 out]
            n264 = property on="In VLV" class="Enum (strict)"("Visible"=w481) -> ()  [unwired: 2 in, 2 out]
            n265 = property on="Drain VLV" class="Enum (strict)"("Visible"=w481) -> ()  [unwired: 2 in, 2 out]
            n266 = property on="Out VLV" class="Enum (strict)"("Visible"=w481) -> ()  [unwired: 2 in, 2 out]
            n267 = case shown="True" w479 {
              tunnel: w481 -> [_ w484]
              tunnel: w480 -> [_ w483]
              frame False {
              }
              frame True {
                n268 = property on="Drain VLV B" class="Enum (strict)"("Visible"=w484) -> ()  [unwired: 2 in, 2 out]
                n269 = property on="Out VLV B" class="Enum (strict)"("Visible"=w484) -> ()  [unwired: 2 in, 2 out]
                n270 = property on="Out VLV C" class="Enum (strict)"("Visible"=w484) -> ()  [unwired: 2 in, 2 out]
                n271 = property on="In VLV B" class="Enum (strict)"("Visible"=w484) -> ()  [unwired: 2 in, 2 out]
                n272 = property on="In VLV C" class="Enum (strict)"("Visible"=w484) -> ()  [unwired: 2 in, 2 out]
                n273 = property on="Drain VLV C" class="Enum (strict)"("Visible"=w484) -> ()  [unwired: 2 in, 2 out]
                n274 = property on="In VLV D" class="Enum (strict)"("Visible"=w484) -> ()  [unwired: 2 in, 2 out]
                n275 = property on="Drain VLV D" class="Enum (strict)"("Visible"=w484) -> ()  [unwired: 2 in, 2 out]
                n276 = property on="Out VLV D" class="Enum (strict)"("Visible"=w484) -> ()  [unwired: 2 in, 2 out]
                n277 = property on="Valve Set B" class="Enum (strict)"("Visible"=w483) -> ()  [unwired: 2 in, 2 out]
                n278 = property on="Valve Set C" class="Enum (strict)"("Visible"=w483) -> ()  [unwired: 2 in, 2 out]
                n279 = property on="Valve Set D" class="Enum (strict)"("Visible"=w483) -> ()  [unwired: 2 in, 2 out]
              }
            }
          }
          event "SetPoint": Value Change {
            n280 = event-data() -> ()  [unwired: 1 in, 5 out]
            n281 = Unbundle By Name(w492) -> ("COM Port"=w488:refnum<visa-resource-name>)
            n282 = flat-sequence {
              tunnel: ["GEA2 Mode Read"] -> w489
              frame #0 {
                "Update Mode" <- TRUE
              }
            }
            n283 = call "HEWH GEA2 Set Tank Mode and Temp.vi"("ComPort"=w488, "Mode"=w489, "Set Point"="SetPoint", "Error In"=w491) -> ("Mode Read"=w486:T7, "SetPoint Read"=w485:u8, "Error Out"=w490:errorcluster)  [unwired: 9 in]
            n284 = local write "SetPoint"(w485) -> ()
            n285 = flat-sequence {
              tunnel: w486 -> [w496]
              frame #0 {
                n286 = local write "GEA2 Mode Read"(w496) -> ()
                n287 = local write "Update Mode"(FALSE ("Update Mode")) -> ()
              }
            }
          }
          event "Drain VLV B", "Out VLV B", "In VLV B": Value Change {
            w499 = u16 1 items=["A", "B", "C", "D"] ("Valve Bank")
            n288 = event-data() -> ()  [unwired: 1 in, 5 out]
            n289 = Unbundle By Name(w501) -> ("MW100"=w500:refnum<visa-resource-name>)
            n290 = local read "Semiphore"() -> (w497:T5)
            n291 = call "Solenoid Bank.vi"("VISA session"=w500, "Semiphore"=w497, "Valve Bank"=w499, "Drain Valve"="Drain VLV B", "Output Valve"="Out VLV B", "Input Valve"="In VLV B") -> ("Error Out"=w498:errorcluster)  [unwired: 8 in, 1 out]
          }
          event "In VLV C", "Out VLV C", "Drain VLV C": Value Change {
            w510 = u16 2 items=["A", "B", "C", "D"] ("Valve Bank")
            n292 = event-data() -> ()  [unwired: 1 in, 5 out]
            n293 = Unbundle By Name(w512) -> ("MW100"=w511:refnum<visa-resource-name>)
            n294 = local read "Semiphore"() -> (w505:T5)
            n295 = call "Solenoid Bank.vi"("VISA session"=w511, "Semiphore"=w505, "Valve Bank"=w510, "Drain Valve"="Drain VLV C", "Output Valve"="Out VLV C", "Input Valve"="In VLV C") -> ("Error Out"=w509:errorcluster)  [unwired: 8 in, 1 out]
          }
          event "In VLV D", "Drain VLV D", "Out VLV D": Value Change {
            w518 = u16 3 items=["A", "B", "C", "D"] ("Valve Bank")
            n296 = event-data() -> ()  [unwired: 1 in, 5 out]
            n297 = Unbundle By Name(w520) -> ("MW100"=w519:refnum<visa-resource-name>)
            n298 = local read "Semiphore"() -> (w513:T5)
            n299 = call "Solenoid Bank.vi"("VISA session"=w519, "Semiphore"=w513, "Valve Bank"=w518, "Drain Valve"="Drain VLV D", "Output Valve"="Out VLV D", "Input Valve"="In VLV D") -> ("Error Out"=w517:errorcluster)  [unwired: 8 in, 1 out]
          }
        }
        n300 = case shown="True" "Read Flow" {
          tunnel: w323 -> [_ w350]
          tunnel: w324 -> [_ w348]
          tunnel: [w330 w346] -> w326
          tunnel: w325 -> [w330 w345]
          frame False {
          }
          frame True {
            w336 = T10 36 items=["4-20_OUT", "Pres_HI1", "Pres_HI2", "Pres_LOW", "Pres_PIN", "HEATER_TOP", "HEATER_BOT", "T_Shell", "FLOWMETER", "WATT_SENSE", "WH_TICK", "Tc_1", "Tc_2", "Tc_3", "Tc_4", "Tc_5", "Tc_6", "Tc_down", "T_Shell_2", "T_Shell_3", "T_Shell_4", "RTD_IN", "RTD_OUT", "RTD_AMB", "INTF_TEMPFLO", "INTF_READY", "INTF_START", "INTF_STOP", "DRM_LOW", "DRM_HIGH", "PWR_MAIN", "VLV_DUMP", "VLV_OUT", "VLV_IN", "WATT_HOURS", "FLOW(SAMPLE)", "GALLONS", "FLOW(GPM)"] ("Channel_Enum")
            w341 = T10 37 items=["4-20_OUT", "Pres_HI1", "Pres_HI2", "Pres_LOW", "Pres_PIN", "HEATER_TOP", "HEATER_BOT", "T_Shell", "FLOWMETER", "WATT_SENSE", "WH_TICK", "Tc_1", "Tc_2", "Tc_3", "Tc_4", "Tc_5", "Tc_6", "Tc_down", "T_Shell_2", "T_Shell_3", "T_Shell_4", "RTD_IN", "RTD_OUT", "RTD_AMB", "INTF_TEMPFLO", "INTF_READY", "INTF_START", "INTF_STOP", "DRM_LOW", "DRM_HIGH", "PWR_MAIN", "VLV_DUMP", "VLV_OUT", "VLV_IN", "WATT_HOURS", "FLOW(SAMPLE)", "GALLONS", "FLOW(GPM)"] ("Channel_Enum")
            n301 = local read "Semiphore"() -> (w337:T5)
            n302 = Unbundle By Name(w350) -> ("MW100"=w349:refnum<visa-resource-name>)
            n303 = call "YKMW100 Receive String-clear buff.vi"("VISA session"=w349, "Semiphore"=w337, "error in (no error)"=w348) -> ("dup VISA session"=w338:refnum<visa-resource-name>, "Read Buffer"=w344:string, "error out"=w347:errorcluster)  [unwired: 10 in]
            n304 = String Length(string=w344) -> (length=w343:i32)
            n305 = Greater Than 0?(x=w343) -> (x > 0?=w342:bool)
            n306 = call "Generic - AI1.vi"("MW100"=w338, "Semiphore"=w337, "Channel_Enum"=w341, "Error In"=w347) -> ("Value"=→"Flow Meter":dbl, "Error Out"=w339:errorcluster)  [unwired: 9 in, 1 out]
            n307 = case shown="False" w342 {
              tunnel: w344 -> [_ w355]
              tunnel: [w351 w353] -> w346
              tunnel: w345 -> [w351 w354]
              frame False {
              }
              frame True {
                # "Bug Chasing.."
                n308 = Build Array (concatenate)(w354, w355) -> (w353:string[])
                "BUG array" <- w353
                n309 = property on="BUG array" class="Arr (strict)"("Visible"=TRUE) -> ()  [unwired: 2 in, 2 out]
              }
            }
            n310 = call "Generic - AI1.vi"("MW100"=w338, "Semiphore"=w337, "Channel_Enum"=w336, "Error In"=w339) -> ("Value"=w332:dbl, "Error Out"=w331:errorcluster)  [unwired: 9 in, 1 out]
            "Gallons" <- w332
            n311 = local write "Error Out"(w331) -> ()
            n312 = call "Calculate_T_to_H2O_LBSperGAL.vi"("Termperature"="Termperature") -> ("lbs/Gal"=w333:dbl)  [unwired: 10 in]
            n313 = Multiply(x=w333, y=w332) -> (x*y=→"LBS":dbl)
          }
        }
        n314 = Unbundle By Name(w322) -> ()  [unwired: 1 out]
        n315 = local write "Error Out"(w322) -> ()
        n316 = Wait (ms)(milliseconds to wait=u32 250) -> ()  [unwired: 1 out]
        "Pulse" <- w327
      }
      n317 = while {
        tunnel: w203 -> [w213]
        stop <- w216 stop-if-true
        n318 = local read "Ready"() -> (w214:bool)
        n319 = case shown="True" w214 {
          tunnel: w213 -> [_ w217]
          tunnel: "GEA2 Max Retry" -> [_ w219]
          tunnel: 1 ("f") -> [_ w218]
          frame False {
          }
          frame True {
            n320 = local read "COM Port"() -> (w221:refnum<visa-resource-name>)
            n321 = Select(t=w219, s=w217, f=w218) -> (s? t:f=w220:i32)
            n322 = call "HEWH Serial Data Read.vi"("Serial Port Ref"=w221, "GEA2 HyperData"=w217, "Retries"=w220) -> ("Read String"=w223:string, "error out"=w222:errorcluster)  [unwired: 9 in, 2 out]
            "Serial Port Error" <- w222
            n323 = case shown="No Error" w222 {
              frame No Error {
                n324 = local write "Serial Port Available?"(TRUE ("Serial Port Available?")) -> ()
              }
              frame Error {
                "Serial Port Available?" <- FALSE ("Gather Data")
              }
            }
            n325 = local write "Serial Data In"(w223) -> ()
          }
        }
        n326 = Wait (ms)(milliseconds to wait=u32 500) -> ()  [unwired: 1 out]
        n327 = local read "Stop Test"() -> (w216:bool)
      }
      n328 = while {
        tunnel: w208 -> [w242]
        shift-right: [w241] -> _
        shift-left: 0 -> [w240]
        shift-right: [w239] -> _
        shift-left: 0.0 -> [w238]
        stop <- w243 stop-if-true
        n329 = case shown="True" TRUE ("Gather Data") {
          tunnel: w242 -> [_ w264]
          tunnel: w240 -> [w246 w254]
          tunnel: [w246 w262] -> w241
          tunnel: [0.0 w260] -> w239
          tunnel: w238 -> [_ w259]
          frame False {
          }
          frame True {
            n330 = case shown="True" "Reset Count" {
              tunnel: [w265 0] -> w255
              tunnel: w254 -> [w265 _]
              frame False {
              }
              frame True {
                n331 = local write "Reset Count"(FALSE ("Update Count")) -> ()
              }
            }
            n332 = Multiply(x="Sample Period (S)", y=1000.0) -> (x*y=w250:dbl)
            n333 = Multiply(x=w259, y=1000.0) -> (x*y=w249:dbl)
            n334 = Subtract(x=w250, y=w249) -> (x-y=w257:dbl)
            n335 = In Range and Coerce(upper limit=w250, x=w257, lower limit=0.0) -> (coerced(x)=w247:dbl)  [unwired: 1 out]
            n336 = To Long Integer(number=w247) -> (32bit integer=w248:i32)
            n337 = event shown="[0] Timeout" {
              selector: _ -> [_]
              dyn-events: _ -> [_]
              timeout: w248 -> [_]
              tunnel: w264 -> [w295]
              tunnel: "Write To File" -> [w294]
              tunnel: w255 -> [w290]
              tunnel: [w287] -> w262
              tunnel: [w286] -> w261
              event Timeout {
                n338 = event-data() -> ()  [unwired: 1 in, 2 out]
                n339 = flat-sequence {
                  tunnel: [w298] -> w286
                  frame #0 {
                    n340 = call "E-Time.vi"() -> ("Elapsed Time (sec)"=w298:dbl)  [unwired: 9 in, 2 out]
                  }
                }
                n341 = local read "Chanel List"() -> (w285:string)
                n342 = local read "Semiphore"() -> (w297:T5)
                n343 = local read "Use Agilent?"() -> (w283:bool)
                n344 = local read "Label Array"() -> (w284:string[])
                n345 = control-ref of="Tank Display"() -> (w296:refnum<vi>)
                n346 = Equal To 0?(x=w290) -> (x = 0?=w292:bool)
                "Header?" <- w292
                n347 = call "Gather Test Data - Heatup Test new.vi"("Agilent Scan List"=w285, "Semiphore"=w297, "Equipment"=w295, "Tank Display Ref"=w296, "Agilent?"=w283, "Serial Data In"="Serial Data In", "Agilent Label Array"=w284) -> ("Output Data"=w281:string[][], "POWER"=→"POWER":T8, "Voltage"=→"Voltage Reading":dbl, "error out"=w291:errorcluster)  [unwired: 3 in, 2 out]
                "Gather Data Error" <- w291
                n348 = local read "file path (dialog if empty)"() -> (w293:path)
                n349 = case shown="True" w294 {
                  tunnel: w281 -> [_ w306]
                  tunnel: w293 -> [_ w305]
                  tunnel: w292 -> [_ w304]
                  tunnel: w290 -> [w300 w302]
                  tunnel: [w300 w303] -> w287
                  frame False {
                  }
                  frame True {
                    n350 = Increment(x=w302) -> (x+1=w301:i32)
                    n351 = case shown="True" w304 {
                      tunnel: w306 -> [w312 w315]
                      tunnel: w305 -> [w309 w317]
                      tunnel: w301 -> [w307 w313]
                      tunnel: [w307 w313] -> w303
                      frame True {
                        n352 = call-poly <vilib>:"Write To Spreadsheet File.vi"("delimiter (\\t)"="," ("delimiter (\\t)"), "append to file? (new file:F)"=TRUE, "2D data"=w312, "file path (dialog if empty)"=w309) -> ()  [unwired: 4 in, 1 out]
                        n353 = local write "Header?"(FALSE ("First Data?")) -> ()
                      }
                      frame False {
                        n354 = Index Array(array=w315, index (row)=1) -> (element=w314:string[])  [unwired: 1 in]
                        n355 = call-poly <vilib>:"Write To Spreadsheet File.vi"("delimiter (\\t)"="," ("delimiter (\\t)"), "append to file? (new file:F)"=TRUE, "1D data"=w314, "file path (dialog if empty)"=w317) -> ()  [unwired: 4 in, 1 out]
                      }
                    }
                  }
                }
                n356 = Transpose 2D Array(2D array=w281) -> (transposed array=w275:string[][])
                n357 = local read "Source Array"() -> (w274:string[])
                n358 = Index Array(array=w275, index (col) #1=0 ("disabled index (col)"), index (col) #2=1 ("index (col)")) -> (element #1=w278:string[], element #2=w279:string[])  [unwired: 2 in]
                n359 = Build Array(w278, w279, w274) -> (w280:string[][])
                n360 = Transpose 2D Array(2D array=w280) -> (transposed array=w271:string[][])
                "DATA - Label, Value, Source" <- w271
                n361 = call "Array_Search_For_Num.vi"("N Rows of Data"=w271, "Title?"="WATT_SENSE") -> ("number"=→"kW":dbl)  [unwired: 12 in, 1 out]
                n362 = case shown="Error" w291 {
                  frame No Error {
                  }
                  frame Error {
                    n363 = call "Delay mS.vi"("milliseconds to wait"=u32 5000) -> ()  [unwired: 14 in, 1 out]
                  }
                }
                "WriteDataCount" <- w290
              }
            }
            n364 = flat-sequence {
              tunnel: w261 -> [w269]
              tunnel: [w268] -> w260
              frame #0 {
                n365 = call "E-Time.vi"() -> ("Elapsed Time (sec)"=w270:dbl)  [unwired: 9 in, 2 out]
                n366 = Subtract(x=w270, y=w269) -> (x-y=w268:dbl)
              }
            }
          }
        }
        n367 = local read "Stop Test"() -> (w243:bool)
      }
    }
    frame Error {
      w521 = TRUE ("Stop Test")
      n368 = local write "Stop Test"(w521) -> ()
      n369 = property on="Stop Test" class="Bool (strict)"("Val(Sgnl)"=w521) -> ()  [unwired: 2 in, 2 out]
    }
  }
  "Error Out" <- w3
  n370 = while {
    stop <- FALSE stop-if-true
    n371 = event shown="[1] \"Stop Test\": Value Change" {
      selector: _ -> [_ _ _ _]
      dyn-events: _ -> [_ _ _ _]
      timeout: _ -> [_ _ _ _]
      event Timeout {
        n372 = event-data() -> ()  [unwired: 1 in, 2 out]
      }
      event "Stop Test": Value Change {
        n373 = event-data() -> ()  [unwired: 1 in, 5 out]
        n374 = local read "Stop Test"() -> (w525:bool)
        n375 = case shown="True" w525 {
          frame False {
          }
          frame True {
            n376 = stacked-sequence {
              frame #0 {
                n377 = local read "MW100"() -> (w529:refnum<visa-resource-name>)
                n378 = local read "Semiphore"() -> (w528:T5)
                n379 = call "Intellifaucet_Driver.vi"("VISA session"=w529, "Mode"=Intellfaucet_Mode."Stop Flow", "Semiphore"=w528) -> ("VISA session out"=w531:refnum<visa-resource-name>, "Error Out"=w535:errorcluster)  [unwired: 11 in]
                n380 = call "Solenoid - Fill.vi"("Semiphore"=w528, "Error In"=w535, "VALVE OPEN CLOSE"=enum8{"OPEN", "CLOSE"}."CLOSE", "VISA session"=w531) -> ("Error Out"=w533:errorcluster, "dup VISA session"=w530:refnum<visa-resource-name>)  [unwired: 6 in]
                n381 = call "Solenoid - DRAIN.vi"("Semiphore"=w528, "Error In"=w533, "VALVE OPEN CLOSE"=enum8{"OPEN", "CLOSE"}."CLOSE", "VISA session"=w530) -> ("Error Out"=→"Stop Err":errorcluster)  [unwired: 6 in, 1 out]
              }
              frame #1 {
                n382 = local read "Equipment"() -> (w539:T4)
                n383 = local read "Semiphore"() -> (w538:T5)
                n384 = call "HEWH CloseEquipmet.vi"("Semiphore"=w538, "Equipment"=w539) -> ("Error Out"=w537:errorcluster)  [unwired: 9 in]
                n385 = local read "Local?"() -> (w536:bool)
                n386 = call "Semiphore-Destroy-Local.vi"("Semiphore"=w538, "Local?"=w536, "error in (no error)"=w537) -> ()  [unwired: 16 in, 1 out]
              }
              frame #2 {
                n387 = local write "Stop Test"(FALSE ("stop")) -> ()
              }
              frame #3 {
                n388 = Stop(stop? (T)=TRUE) -> ()
              }
            }
          }
        }
      }
      event "P-H": Value Change {
        n389 = event-data() -> ()  [unwired: 1 in, 5 out]
        n390 = local read "DATA - Label, Value, Source"() -> (w542:string[][])
        n391 = Transpose 2D Array(2D array=w542) -> (transposed array=w543:string[][])
        n392 = stacked-sequence {
          tunnel: w543 -> [w555 w558 w561 w564 w567 w570]
          tunnel: [w553 _ _ _ _ _] -> w551
          tunnel: [_ w556 _ _ _ _] -> w550
          tunnel: [_ _ w559 _ _ _] -> w549
          tunnel: [_ _ _ w562 _ _] -> w548
          tunnel: [_ _ _ _ w565 _] -> w547
          tunnel: [_ _ _ _ _ w568] -> w546
          tunnel: "P-H" -> [_ _ _ _ _ _]
          frame #0 {
            n393 = call "Array_Search_For_Num.vi"("N Rows of Data"=w555, "Title?"="Pres_HI1 (P1)") -> ("number"=w553:dbl)  [unwired: 12 in, 1 out]
          }
          frame #1 {
            n394 = call "Array_Search_For_Num.vi"("N Rows of Data"=w558, "Title?"="Pres_LOW (P3)") -> ("number"=w556:dbl)  [unwired: 12 in, 1 out]
          }
          frame #2 {
            n395 = call "Array_Search_For_Num.vi"("N Rows of Data"=w561, "Title?"="Pres_HI2 (P2)") -> ("number"=w559:dbl)  [unwired: 12 in, 1 out]
          }
          frame #3 {
            n396 = call "Array_Search_For_Num.vi"("N Rows of Data"=w564, "Title?"="T3B(EvapOut)") -> ("number"=w562:dbl)  [unwired: 12 in, 1 out]
          }
          frame #4 {
            n397 = call "Array_Search_For_Num.vi"("N Rows of Data"=w567, "Title?"="T4(CompressorDischarge)") -> ("number"=w565:dbl)  [unwired: 12 in, 1 out]
          }
          frame #5 {
            n398 = call "Array_Search_For_Num.vi"("N Rows of Data"=w570, "Title?"="T3A(EvapIn)") -> ("number"=w568:dbl)  [unwired: 12 in, 1 out]
          }
        }
        n399 = call "R134a-PH Curves.vi"("P1 (Compressor In, P Low)"=w550, "P2 (Compressor Out, P High1)"=w551, "P5 (Expansion In, P High2)"=w549, "T1 (Compressor In, T3B)"=w548, "T2 Compressor Out, T4)"=w547, "T6 (Evap In, T3A)"=w546) -> ("P-T-H Data"=w544:dbl[][])  [unwired: 8 in, 1 out]
        n400 = flat-sequence {
          tunnel: w544 -> [_]
          frame #0 {
            n401 = local write "P-H"(FALSE ("P-H")) -> ()
          }
        }
      }
      event "Help": Value Change {
        n402 = event-data() -> ()  [unwired: 1 in, 5 out]
        n403 = One Button Dialog(message="This program is intended to be used to manually control the HEWH test stand.  It allows independant control of all of the IO used in the DOE test.  It allows you to gather and save test data, even if the serial port is not available every 10 seconds..") -> (true=w572:bool)  [unwired: 1 in]
        n404 = Not(x=w572) -> (.not. x?=w571:bool)
        n405 = local write "Help"(w571) -> ()
      }
    }
    n406 = Wait (ms)(milliseconds to wait=u32 250) -> ()  [unwired: 1 out]
  }
